vi "to string.vi"(8 "error in":errorcluster, 11 "Profibus Module configuration in":refnum<class "Profibus Module configuration.lvclass">) -> (0 "error out":errorcluster, 1 "data":string, 2 "version":string, 3 "Profibus Module configuration out":refnum<class "Profibus Module configuration.lvclass">)   [LabVIEW 2013, in "Profibus Module configuration.lvclass"]
doc: "Provides an interface for saving a module configuration to a file or other serialized data source. It is recommended that all children of this class store data in two sets--data required for its own initialization, and any data required for parent initialization--and that each implementation uses the <b>Call Parent Method</b> primitive to serialize parent information."
uses:
  Profibus Module configuration.lvclass
  <vilib>/NI/Tag Bus Module Framework/module configuration/TBM module configuration.lvclass
  Profibus Module configuration.lvclass/Profibus Module configuration.ctl
  current version.vi
  <vilib>/NI/Tag Bus Module Framework/root configuration/TBM configuration.lvclass
  channel/Profibus channel.lvclass
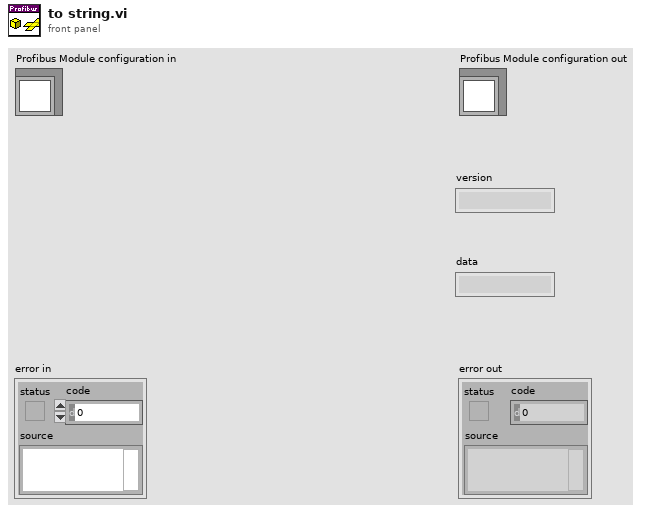
[diagram p1: front panel]
types:
  T1 = typedef "Profibus Module configuration.lvclass/endianness setting.ctl" = cluster{"slave":i8, "big endian":bool}
  T2 = typedef "Profibus Module configuration.lvclass/slave diagnostic configuration.ctl" = cluster{"slave":i8, "report":bool, "channel":refnum<class "TBM channel.lvclass">, "error specs":T3[]}
  T3 = typedef "Profibus Module configuration.lvclass/error throw specification.ctl" = cluster{"byte":i32, "bit":i32, "inverted?":bool, "error":i32}
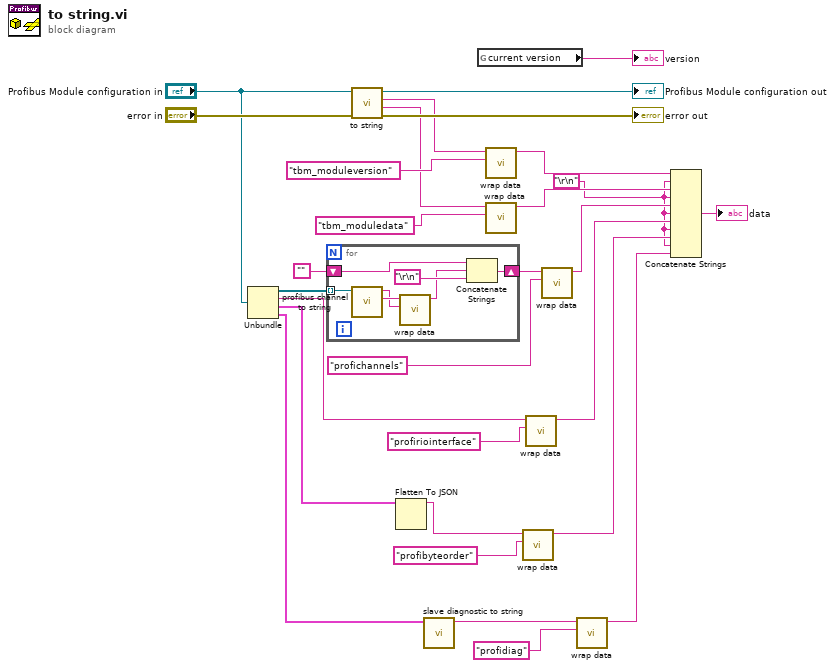
[diagram p0: block diagram]
diagram:
  w3 = "\r\n"
  n1 = Unbundle("Profibus Module configuration in") -> (w15:refnum<class "Profibus channel.lvclass">[], w10:string, w9:T1[], w5:T2[])
  n2 = for {
    tunnel: w15 -> [w36] mode=indexing
    shift-right: [w32] -> w13
    shift-left: "" -> [w31]
    n3 = call "profibus channel to string.vi"("Profibus channel in"=w36) -> ("channel data"=w35:string, "identifier"=w34:string)  [unwired: 9 in]
    n4 = call <vilib>:"wrap data.vi"("identifier"=w34, "data to wrap"=w35) -> ("wrapped data"=w30:string)  [unwired: 9 in]
    n5 = Concatenate Strings(w31, w30, "\r\n") -> (w32:string)
  }
  n6 = call-parent "to string.vi"("error in"="error in", "module configuration in"="Profibus Module configuration in") -> ("error out"=→"error out":errorcluster, "data"=w20:string, "version"=w21:string, "module configuration out"=→"Profibus Module configuration out":refnum<class "Profibus Module configuration.lvclass">)  [unwired: 6 in]
  n7 = Flatten To JSON(anything=w9) -> (JSON string=w7:string)  [unwired: 2 in, 1 out]
  n8 = call "slave diagnostic to string.vi"("slave diagnostics"=w5) -> ("data string"=w4:string)  [unwired: 10 in]
  n9 = global read "current version.vi" "current version"() -> (→"version":string)
  n10 = call <vilib>:"wrap data.vi"("identifier"="tbm_moduleversion" ("additional identifier"), "data to wrap"=w21) -> ("wrapped data"=w23:string)  [unwired: 9 in]
  n11 = call <vilib>:"wrap data.vi"("identifier"="tbm_moduledata" ("additional identifier"), "data to wrap"=w20) -> ("wrapped data"=w22:string)  [unwired: 9 in]
  n12 = call <vilib>:"wrap data.vi"("identifier"="profibyteorder" ("additional identifier"), "data to wrap"=w7) -> ("wrapped data"=w6:string)  [unwired: 9 in]
  n13 = call <vilib>:"wrap data.vi"("identifier"="profiriointerface" ("additional identifier"), "data to wrap"=w10) -> ("wrapped data"=w12:string)  [unwired: 9 in]
  n14 = call <vilib>:"wrap data.vi"("identifier"="profichannels" ("additional identifier"), "data to wrap"=w13) -> ("wrapped data"=w17:string)  [unwired: 9 in]
  n15 = call <vilib>:"wrap data.vi"("identifier"="profidiag", "data to wrap"=w4) -> ("wrapped data"=w2:string)  [unwired: 9 in]
  n16 = Concatenate Strings(w23, w3, w22, w3, w17, w3, w12, w3, w6, w3, w2) -> (→"data":string)
